vi "Build Sim Device List_ALT.vi"() -> (3 "Sim Device List":T1)   [LabVIEW 2019]
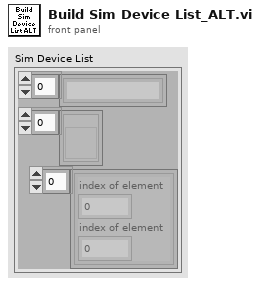
[diagram p1: front panel]
types:
  T1 = cluster{string[], refnum<vi>[], cluster{"index of element":i32, "index of element":i32}[]}
  T2 = cluster{string[], refnum<vi>[], cluster{i32, i32}[]}
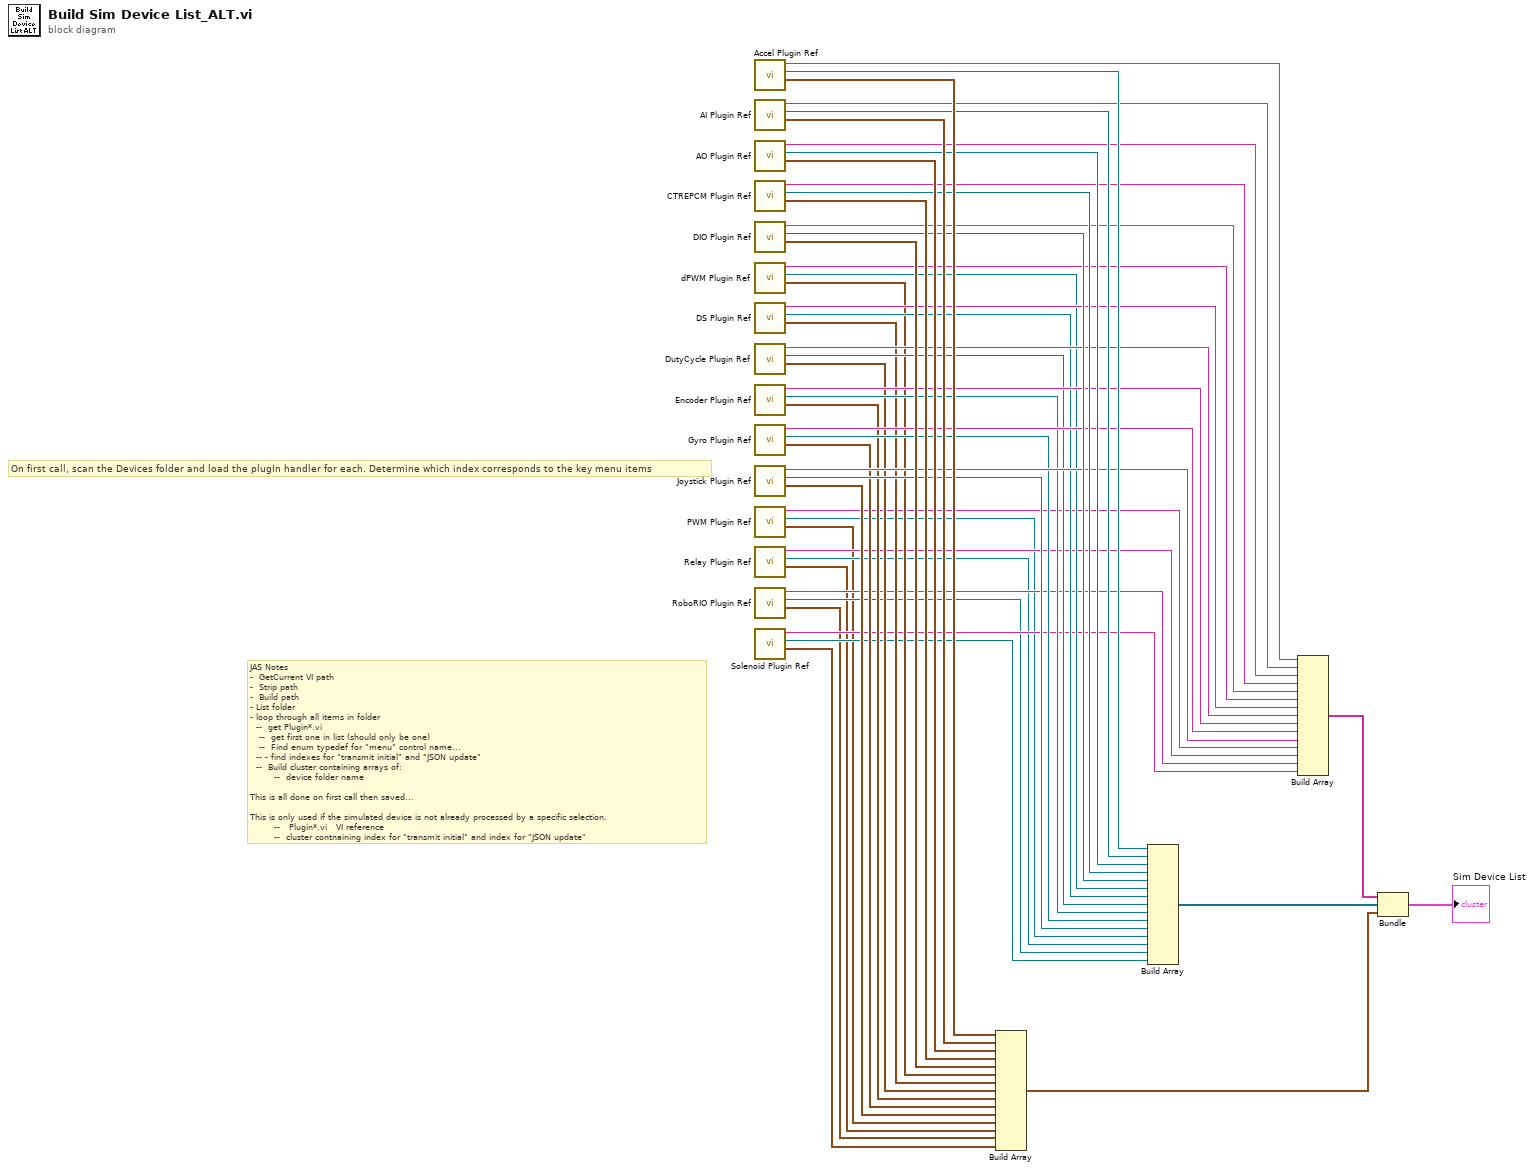
[diagram p0: block diagram]
diagram:
  # "JAS Notes\n-  GetCurrent VI path\n-  Strip path\n-  Build path\n- List folder\n- loop through all items in folder\n  --  get Plugin*.vi\n   --  get first one in list (should only be one)\n   --  Find enum typedef for \"menu\" control name... \n  -- - find indexes for \"transmit initial\" and \"JSON update\"\n  --  Build cluster containing arrays of:\n        --  device folder name\n\nThis is all done on first call then saved...\n\nThis is only used if the simulated device is not already processed by a specific selection.\n        --   Plugin*.vi   VI reference\n        --  cluster contnaining index for \"transmit initial\" and index for \"JSON update\""
  # "On first call, scan the Devices folder and load the plugIn handler for each. Determine which index corresponds to the key menu items"
  n1 = call "Accel Plugin Ref.vi"() -> ("Command Index"=w44:cluster{i32, i32}, "Plugin VI Ref"=w45:refnum<vi>, "Device Type"=w46:string)  [unwired: 9 in]
  n2 = call "AI Plugin Ref.vi"() -> ("Command Index"=w41:cluster{i32, i32}, "Plugin VI Ref"=w42:refnum<vi>, "Device Type"=w43:string)  [unwired: 9 in]
  n3 = call "AO Plugin Ref.vi"() -> ("Command Index"=w38:cluster{i32, i32}, "Plugin VI Ref"=w39:refnum<vi>, "Device Type"=w40:string)  [unwired: 9 in]
  n4 = call "CTREPCM Plugin Ref.vi"() -> ("Command Index"=w35:cluster{i32, i32}, "Plugin VI Ref"=w36:refnum<vi>, "Device Type"=w37:string)  [unwired: 9 in]
  n5 = call "DIO Plugin Ref.vi"() -> ("Command Index"=w32:cluster{i32, i32}, "Plugin VI Ref"=w33:refnum<vi>, "Device Type"=w34:string)  [unwired: 9 in]
  n6 = call "dPWM Plugin Ref.vi"() -> ("Command Index"=w18:cluster{i32, i32}, "Plugin VI Ref"=w24:refnum<vi>, "Device Type"=w31:string)  [unwired: 9 in]
  n7 = call "DS Plugin Ref.vi"() -> ("Command Index"=w17:cluster{i32, i32}, "Plugin VI Ref"=w23:refnum<vi>, "Device Type"=w30:string)  [unwired: 9 in]
  n8 = call "DutyCycle Plugin Ref.vi"() -> ("Command Index"=w16:cluster{i32, i32}, "Plugin VI Ref"=w22:refnum<vi>, "Device Type"=w29:string)  [unwired: 9 in]
  n9 = call "Encoder Plugin Ref.vi"() -> ("Command Index"=w15:cluster{i32, i32}, "Plugin VI Ref"=w21:refnum<vi>, "Device Type"=w27:string)  [unwired: 9 in]
  n10 = call "Gyro Plugin Ref.vi"() -> ("Command Index"=w14:cluster{i32, i32}, "Plugin VI Ref"=w20:refnum<vi>, "Device Type"=w26:string)  [unwired: 9 in]
  n11 = call "Joystick Plugin Ref.vi"() -> ("Command Index"=w13:cluster{i32, i32}, "Plugin VI Ref"=w19:refnum<vi>, "Device Type"=w25:string)  [unwired: 9 in]
  n12 = call "PWM Plugin Ref.vi"() -> ("Command Index"=w4:cluster{i32, i32}, "Plugin VI Ref"=w8:refnum<vi>, "Device Type"=w12:string)  [unwired: 9 in]
  n13 = call "Relay Plugin Ref.vi"() -> ("Command Index"=w3:cluster{i32, i32}, "Plugin VI Ref"=w7:refnum<vi>, "Device Type"=w11:string)  [unwired: 9 in]
  n14 = call "RoboRIO Plugin Ref.vi"() -> ("Command Index"=w2:cluster{i32, i32}, "Plugin VI Ref"=w6:refnum<vi>, "Device Type"=w10:string)  [unwired: 9 in]
  n15 = call "Solenoid Plugin Ref.vi"() -> ("Command Index"=w1:cluster{i32, i32}, "Plugin VI Ref"=w5:refnum<vi>, "Device Type"=w9:string)  [unwired: 9 in]
  n16 = Build Array(w44, w41, w38, w35, w32, w18, w17, w16, w15, w14, w13, w4, w3, w2, w1) -> (w47:cluster{i32, i32}[])
  n17 = Build Array(w45, w42, w39, w36, w33, w24, w23, w22, w21, w20, w19, w8, w7, w6, w5) -> (w48:refnum<vi>[])
  n18 = Build Array(w46, w43, w40, w37, w34, w31, w30, w29, w27, w26, w25, w12, w11, w10, w9) -> (w28:string[])
  n19 = Bundle(w28, w48, w47) -> (→"Sim Device List":T2)  [unwired: 1 in]
